vi "Enable DQMH Version Caracteristics.vi"(11 "Ctl Array":refnum<vi>[](array[refnum])) -> ()   [LabVIEW 2019, in "Panther Dashboard.lvlib"]
uses:
  Panther Dashboard.lvlib
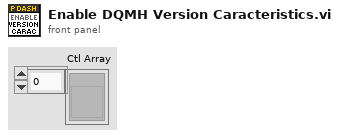
[diagram p1: front panel]
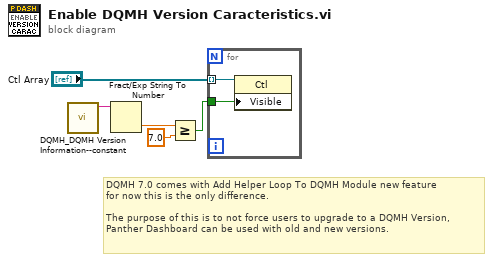
[diagram p0: block diagram]
diagram:
  # "DQMH 7.0 comes with Add Helper Loop To DQMH Module new feature\nfor now this is the only difference.\n\nThe purpose of this is to not force users to upgrade to a DQMH Version,\nPanther Dashboard can be used with old and new versions."
  n1 = call <vilib>:"DQMH_DQMH Version Information--constant.vi"() -> ("DQMH Version"=w3:string)  [unwired: 11 in]
  n2 = Fract/Exp String To Number(string=w3) -> (number=w4:dbl)  [unwired: 3 in, 1 out]
  n3 = Greater Or Equal?(x=w4, y=7.0) -> (x >= y?=w1:bool)
  n4 = for {
    tunnel: "Ctl Array" -> [w7] mode=indexing
    tunnel: w1 -> [w6]
    n5 = property class="Ctl"(reference=w7, "Visible"=w6) -> ()  [unwired: 1 in, 2 out]
  }
